vi "ConfigAndGrabEdited.vi"() -> ()   [LabVIEW 2025]
uses:
  <vilib>/vision/driver/NI_Vision_Acquisition_Software.lvlib
  <resource>/objmgr/imaqdx.rc
  <vilib>/vision/driver/IMAQdx.llb/IMAQdx Buffer Number Mode.ctl
  <vilib>/httpClient/LabVIEWHTTPClient.lvlib
  <vilib>/userDefined/High Color/IMAQdx.ctl
panel:
  in  "URL adress of the backend":string
  out "body":string
  out "error out":errorcluster
  in  "Packet size":i64=1 min=1 step=1
  out "DeviceModelName":string
  in  "OffsetY":i64=100
  in  "Height":i64=600 min=1 max=1088 step=1
  in  "OffsetX":i64=200
  in  "Width":i64=800 min=1 max=2048 step=1
  in  "ExposureTime":dbl=850.5 min=0.0 format="%#_9f"
  in  "Camera Name":T1
  out "Frame Rate":dbl(knob) scale=0.0..100.0 scale format="%.1f"
  out "Buffer Number":u32
  out "Image":T2(plugin-control)
  in  "stop":bool
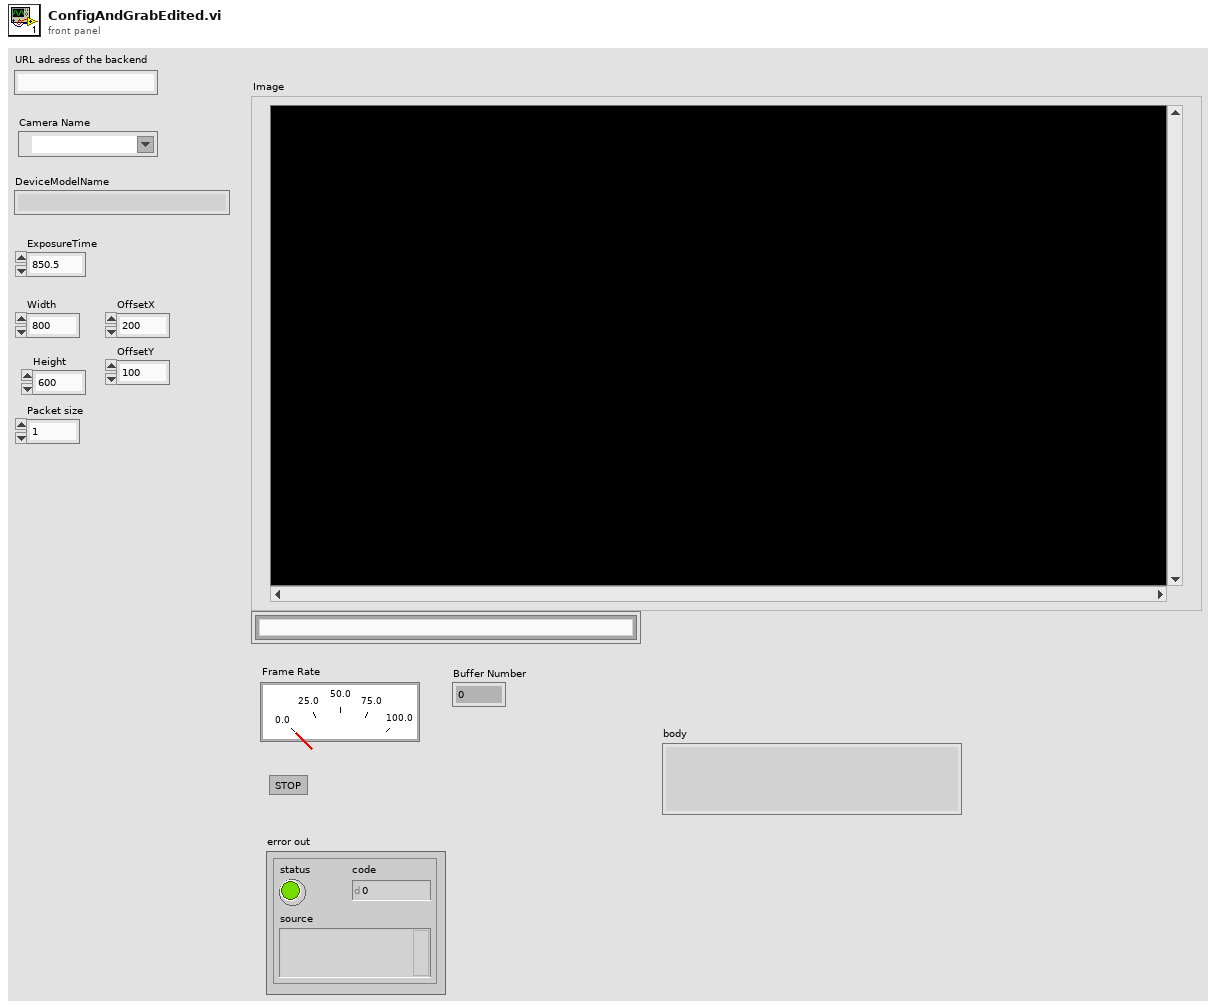
[diagram p1: front panel]
types:
  T1 = typedef "IMAQdx.ctl" = refnum<k21>
  T2 = typedef "IMAQ Image.ctl" = refnum<image>
  T3 = typedef "NI_Vision_Acquisition_Software.lvlib/IMAQdx Buffer Number Mode.ctl" = enum32{"Next", "Last", "Buffer Number", "Every", "Last New"}
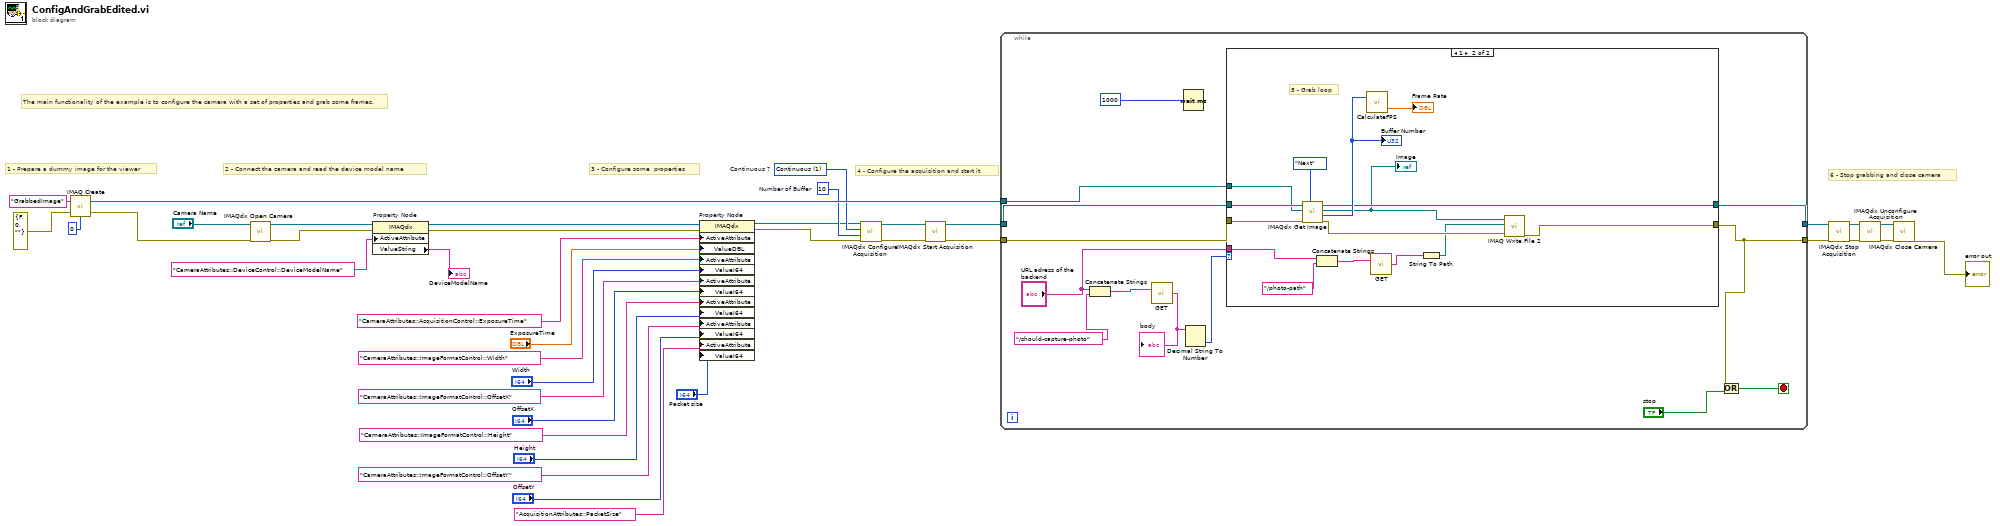
[diagram p0: block diagram]
diagram:
  w22 = u32 10  # Number of Buffer
  w21 = u32 1 items=["One Shot", "Continuous"]  # Continuous ?
  # "The main functionality of the example is to configure the camera with a set of properties and grab some frames."
  # "6 - Stop grabbing and close camera"
  # "4 - Configure the acquisition and start it"
  # "3 - Configure some  properties"
  # "2 - Connect the camera and read the device model name"
  # "1 - Prepare a dummy image for the viewer"
  n1 = call "IMAQ Create"("Image Name"="GrabbedImage", "Image Type"=0, "error in (no error)"=errorcluster {"status"=FALSE, "code"=0, "source"=""}) -> ("New Image"=w25:T2, "error out"=w26:errorcluster)  [unwired: 1 in, 1 out]
  n2 = call <vilib>:"IMAQdx Open Camera.vi"("error in"=w26, "Session In"="Camera Name") -> ("error out"=w7:errorcluster, "Session Out"=w23:T1)  [unwired: 8 in]
  n3 = property on="Property Node" class="IMAQdx"(reference=w23, error in=w7, "ActiveAttribute"="CameraAttributes::DeviceControl::DeviceModelName") -> (reference out=w8:T1, error out=w6:errorcluster, "ValueString"=→"DeviceModelName":string)
  n4 = property on="Property Node" class="IMAQdx"(reference=w8, error in=w6, "ActiveAttribute"="CameraAttributes::AcquisitionControl::ExposureTime", "ValueDBL"="ExposureTime", "ActiveAttribute"="CameraAttributes::ImageFormatControl::Width", "ValueI64"="Width", "ActiveAttribute"="CameraAttributes::ImageFormatControl::OffsetX", "ValueI64"="OffsetX", "ActiveAttribute"="CameraAttributes::ImageFormatControl::Height", "ValueI64"="Height", "ActiveAttribute"="CameraAttributes::ImageFormatControl::OffsetY", "ValueI64"="OffsetY", "ActiveAttribute"="AcquisitionAttributes::PacketSize", "ValueI64"="Packet size") -> (reference out=w20:T1, error out=w19:errorcluster)
  n5 = call <vilib>:"IMAQdx Configure Acquisition.vi"("error in"=w19, "Number of Buffers"=w22, "Continuous?"=w21, "Session In"=w20) -> ("error out"=w39:errorcluster, "Session Out"=w38:T1)  [unwired: 6 out]
  n6 = call <vilib>:"IMAQdx Start Acquisition.vi"("error in"=w39, "Session In"=w38) -> ("error out"=w37:errorcluster, "Session Out"=w36:T1)  [unwired: 8 out]
  n7 = while {
    tunnel: w37 -> [w46]
    tunnel: w36 -> [w52]
    tunnel: w25 -> [w51]
    tunnel: [w45] -> w31
    tunnel: [w50] -> w30
    stop <- w44 stop-if-true
    n8 = Concatenate Strings("URL adress of the backend", "/should-capture-photo" ("string")) -> (w40:string)
    n9 = call <vilib>:"GET.vi"("url"=w40) -> ("body"=w47:string)  [unwired: 11 in, 3 out]
    "body" <- w47
    n10 = Wait (ms)(milliseconds to wait=u32 1000) -> ()  [unwired: 1 out]
    n11 = Decimal String To Number(string=w47) -> (number=w49:i32)  [unwired: 2 in, 1 out]
    n12 = case shown="1" w49 {
      tunnel: w52 -> [w54 w69]
      tunnel: w46 -> [w53 w68]
      tunnel: w51 -> [_ w64]
      tunnel: [w54 w63] -> w50
      tunnel: [w53 w60] -> w45
      tunnel: "URL adress of the backend" -> [_ w58]
      frame 0, Default {
      }
      frame 1 {
        # "5 - Grab loop"
        n13 = call <vilib>:"IMAQdx Get Image.vi"("Buffer Number Mode (Next)"=IMAQdx_Buffer_Number_Mode."Next", "error in"=w68, "Image In"=w64, "Session In"=w69) -> ("error out"=w61:errorcluster, "Buffer Number Out"=w65:u32, "Image Out"=w62:T2, "Session Out"=w63:T1)  [unwired: 4 in]
        "Buffer Number" <- w65
        "Image" <- w62
        n14 = Concatenate Strings(w58, "/photo-path" ("string")) -> (w55:string)
        n15 = call "CalculateFPS.vi"("buffer number"=w65) -> ("processed FPS"=→"Frame Rate":dbl)  [unwired: 2 out]
        n16 = call <vilib>:"GET.vi"("url"=w55) -> ("body"=w57:string)  [unwired: 11 in, 3 out]
        n17 = String To Path(string=w57) -> (path=w56:path)
        n18 = call-poly "IMAQ Write File 2"("error in (no error)"=w61, "File Path"=w56, "Image"=w62) -> ("error out"=w60:errorcluster)  [unwired: 7 in, 1 out]
      }
    }
    n19 = Or(x=w45, y="stop") -> (x .or. y?=w44:bool)
  }
  n20 = call <vilib>:"IMAQdx Stop Acquisition.vi"("error in"=w31, "Session In"=w30) -> ("error out"=w35:errorcluster, "Session Out"=w34:T1)  [unwired: 8 out]
  n21 = call <vilib>:"IMAQdx Unconfigure Acquisition.vi"("error in"=w35, "Session In"=w34) -> ("error out"=w32:errorcluster, "Session Out"=w33:T1)  [unwired: 8 out]
  n22 = call <vilib>:"IMAQdx Close Camera.vi"("error in"=w32, "Session In"=w33) -> ("error out"=→"error out":errorcluster)  [unwired: 9 out]
